vi "MecaWheel_New.vi"(8 "RearRightSpeed":dbl format="%19.3f", 9 "RearLeftSpeed":dbl format="%19.3f", 10 "FrontRightSpeed":dbl format="%19.3f", 11 "FrontLeftSpeed":dbl format="%19.3f") -> (3 "MECA_WHEEL_SPEEDS":T1 {"RearRightSpeed" format="%19.3f"; "RearLeftSpeed" format="%19.3f"; "FrontRightSpeed" format="%19.3f"; "FrontLeftSpeed" format="%19.3f"})   [LabVIEW 2019, in "Trajectory_Library.lvlib"]
doc: "Constructs a MecanumDriveWheelSpeeds data structure.\n\nParameters:\n - Left Front Speed - Speed of left front wheel (meters/sec)\n - Right Front Speed - Speed of right front wheel (meters/sec)\n - Left Rear Speed - Speed of left rear wheel (meters/sec)\n - Right Rear Speed - Speed of right rear wheel (meters/sec)\n\nReturns:\n - Meca_wheel_speeds - Data structure\n - Normalized Right Wheel Demand"
uses:
  Trajectory_Library.lvlib
  TypeDef/MECA_WHEEL_SPEEDS.ctl
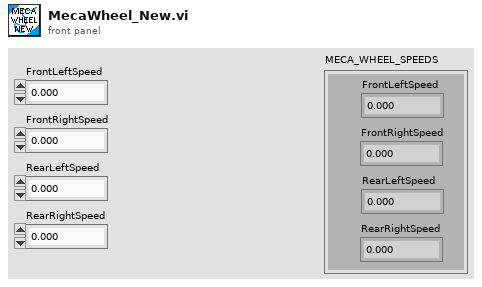
[diagram p1: front panel]
types:
  T1 = typedef "Trajectory_Library.lvlib/MECA_WHEEL_SPEEDS.ctl" = cluster{"FrontLeftSpeed":dbl, "FrontRightSpeed":dbl, "RearLeftSpeed":dbl, "RearRightSpeed":dbl}
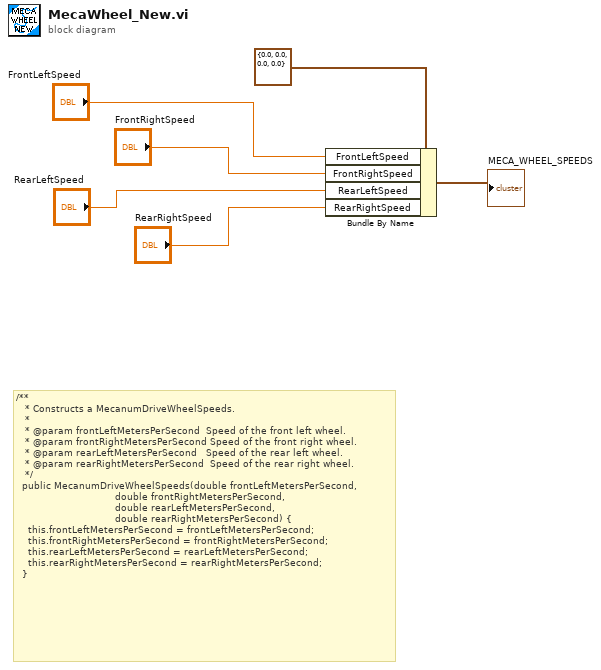
[diagram p0: block diagram]
diagram:
  # "/**\n   * Constructs a MecanumDriveWheelSpeeds.\n   *\n   * @param frontLeftMetersPerSecond  Speed of the front left wheel.\n   * @param frontRightMetersPerSecond Speed of the front right wheel.\n   * @param rearLeftMetersPerSecond   Speed of the rear left wheel.\n   * @param rearRightMetersPerSecond  Speed of the rear right wheel.\n   */\n  public MecanumDriveWheelSpeeds(double frontLeftMetersPerSecond,\n                                 double frontRightMetersPerSecond,\n                                 double rearLeftMetersPerSecond,\n                                 double rearRightMetersPerSecond) {\n    this.frontLeftMetersPerSecond = frontLeftMetersPerSecond;\n    this.frontRightMetersPerSecond = frontRightMetersPerSecond;\n    this.rearLeftMetersPerSecond = rearLeftMetersPerSecond;\n    this.rearRightMetersPerSecond = rearRightMetersPerSecond;\n  }"
  n1 = Bundle By Name(cluster=T1 {"FrontLeftSpeed"=0.0, "FrontRightSpeed"=0.0, "RearLeftSpeed"=0.0, "RearRightSpeed"=0.0} ("MECA_WHEEL_SPEEDS"), "FrontLeftSpeed"="FrontLeftSpeed", "FrontRightSpeed"="FrontRightSpeed", "RearLeftSpeed"="RearLeftSpeed", "RearRightSpeed"="RearRightSpeed") -> (→"MECA_WHEEL_SPEEDS":T1)
